vi "Measurement.WavelengthSweeping.UI.SetDependencies.vi"(8 "error in (no error)":errorcluster, 10 "Dependencies":T1, 11 "Measurement.PhotocurrentMapping.UI in":refnum<class "Measurement.PhotocurrentMapping.UI.lvclass">) -> (0 "error out":errorcluster, 3 "Measurement.PhotocurrentMapping.UI out":refnum<class "Measurement.PhotocurrentMapping.UI.lvclass">)   [LabVIEW 2017, in "Measurement.PhotocurrentMapping.UI.lvclass"]
uses:
  Measurement.PhotocurrentMapping.UI.lvclass
  Typedefs/Dependencies--Cluster.ctl
  Measurement.PhotocurrentMapping/Measurement.PhotocurrentMapping.lvclass
  Measurement.PhotocurrentMapping.UI.lvclass/Measurement.PhotocurrentMapping.UI.ctl
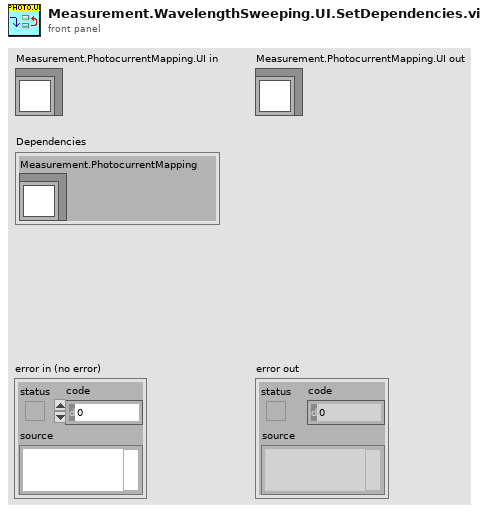
[diagram p1: front panel]
types:
  T1 = typedef "Measurement.PhotocurrentMapping.UI.lvclass/Dependencies--Cluster.ctl" = cluster{"Measurement.PhotocurrentMapping":refnum<class "Measurement.PhotocurrentMapping.lvclass">}
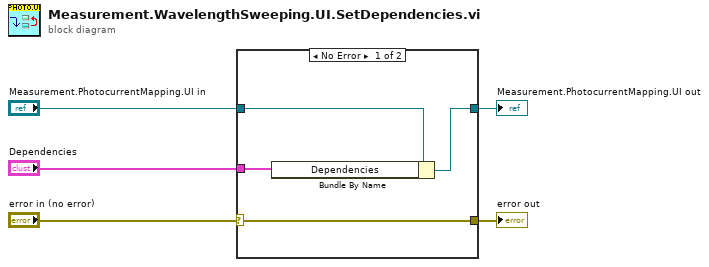
[diagram p0: block diagram]
diagram:
  n1 = case shown="No Error" "error in (no error)" {
    selector: "error in (no error)" -> [w9 w11]
    tunnel: [w9 w11] -> w4
    tunnel: [w6 w10] -> w2
    tunnel: "Measurement.PhotocurrentMapping.UI in" -> [w8 w10]
    tunnel: "Dependencies" -> [w7 _]
    frame No Error {
      n2 = Bundle By Name(cluster=w8, "Dependencies"=w7) -> (w6:refnum<class "Measurement.PhotocurrentMapping.UI.lvclass">)
    }
    frame Error {
    }
  }
  "error out" <- w4
  "Measurement.PhotocurrentMapping.UI out" <- w2
